vi "GetVibrationChannelProperties.vi"(10 "all channels":T2[](array[typedef]), 11 "channel":T2) -> (2 "TDMS properties":T1[](array[typedef]))   [LabVIEW 2017, in "Tdms.lvlib"]
doc: "Returns TDMS properties that define how a waveform channel works. Use the TDMS Set Properties function to write these properties to a TDMS file that contains data from the channel."
uses:
  <vilib>/addons/InsightCM/Utilities/Tdms/Tdms.lvlib
  <vilib>/addons/InsightCM/MessageBus/Base/controls/R2_Channel.ctl
  <vilib>/addons/InsightCM/MessageBus/Base/controls/KeyValuePair.ctl
  <vilib>/addons/InsightCM/MessageBus/Base/controls/Metric.ctl
  <vilib>/addons/InsightCM/Utilities/Tdms/controls/Property.ctl
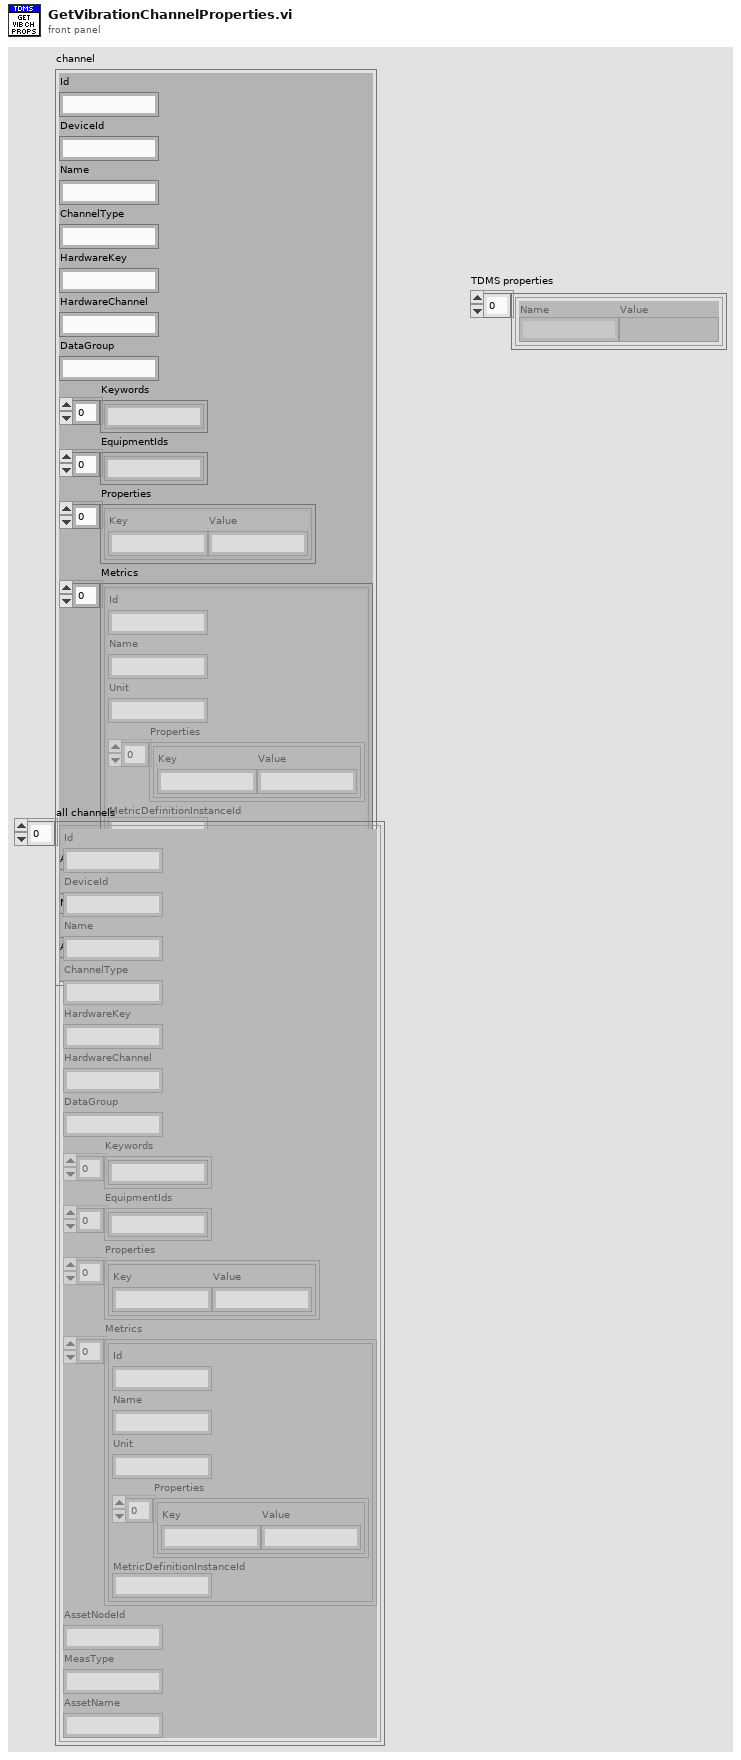
[diagram p1: front panel]
types:
  T1 = typedef "Tdms.lvlib/Property.ctl" = cluster{"Name":string, "Value":variant}
  T2 = typedef "R2_Channel.ctl" = cluster{"Id":string, "DeviceId":string, "Name":string, "ChannelType":string, "HardwareKey":string, "HardwareChannel":string, "DataGroup":string, "Keywords":string[], "EquipmentIds":string[], "Properties":T3[], "Metrics":T4[], "AssetNodeId":string, "MeasType":string, "AssetName":string}
  T3 = typedef "KeyValuePair.ctl" = cluster{"Key":string, "Value":string}
  T4 = typedef "Metric.ctl" = cluster{"Id":string, "Name":string, "Unit":string, "Properties":T3[], "MetricDefinitionInstanceId":string}
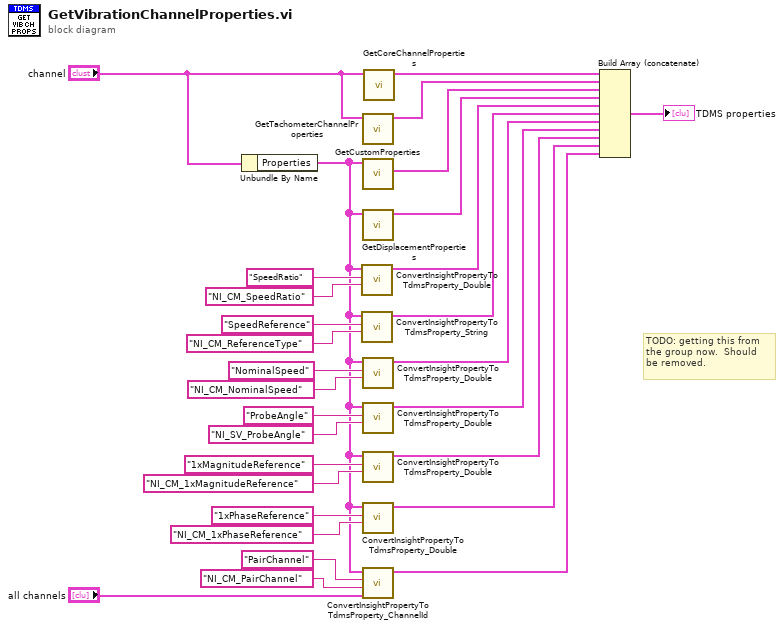
[diagram p0: block diagram]
diagram:
  # "TODO: getting this from\nthe group now.  Should\nbe removed."
  n1 = Unbundle By Name("channel") -> ("Properties"=w3:T3[])
  n2 = call <vilib>:"ConvertInsightPropertyToTdmsProperty_Double.vi"("Tdms Property Name"="NI_CM_SpeedRatio" ("Name"), "Insight Property Name"="SpeedRatio" ("Name"), "Insight Properties"=w3) -> ("Tdms Properties"=w2:T1[])  [unwired: 8 in]
  n3 = call <vilib>:"ConvertInsightPropertyToTdmsProperty_String.vi"("Tdms Property Name"="NI_CM_ReferenceType" ("Name"), "Insight Property Name"="SpeedReference" ("Name"), "Insight Properties"=w3) -> ("Tdms Properties"=w14:T1[])  [unwired: 8 in]
  n4 = call <vilib>:"GetTachometerChannelProperties.vi"("Channel"="channel") -> ("Tachometer Properties"=w7:T1[])  [unwired: 10 in]
  n5 = call <vilib>:"GetCustomProperties.vi"("Properties"=w3) -> ("Tdms Properties"=w6:T1[])  [unwired: 10 in]
  n6 = call <vilib>:"GetDisplacementProperties.vi"("channel properties"=w3) -> ("tdms properties"=w1:T1[])  [unwired: 10 in]
  n7 = call <vilib>:"ConvertInsightPropertyToTdmsProperty_Double.vi"("Tdms Property Name"="NI_CM_NominalSpeed" ("Name"), "Insight Property Name"="NominalSpeed" ("Name"), "Insight Properties"=w3) -> ("Tdms Properties"=w13:T1[])  [unwired: 8 in]
  n8 = call <vilib>:"ConvertInsightPropertyToTdmsProperty_Double.vi"("Tdms Property Name"="NI_SV_ProbeAngle" ("Name"), "Insight Property Name"="ProbeAngle" ("Name"), "Insight Properties"=w3) -> ("Tdms Properties"=w12:T1[])  [unwired: 8 in]
  n9 = call <vilib>:"ConvertInsightPropertyToTdmsProperty_Double.vi"("Tdms Property Name"="NI_CM_1xMagnitudeReference" ("Name"), "Insight Property Name"="1xMagnitudeReference" ("Name"), "Insight Properties"=w3) -> ("Tdms Properties"=w11:T1[])  [unwired: 8 in]
  n10 = call <vilib>:"ConvertInsightPropertyToTdmsProperty_Double.vi"("Tdms Property Name"="NI_CM_1xPhaseReference" ("Name"), "Insight Property Name"="1xPhaseReference" ("Name"), "Insight Properties"=w3) -> ("Tdms Properties"=w10:T1[])  [unwired: 8 in]
  n11 = call <vilib>:"ConvertInsightPropertyToTdmsProperty_ChannelId.vi"("Insight Channels"="all channels", "Tdms Property Name"="NI_CM_PairChannel" ("Name"), "Insight Property Name"="PairChannel" ("Name"), "Insight Properties"=w3) -> ("Tdms Properties"=w4:T1[])  [unwired: 7 in]
  n12 = call <vilib>:"GetCoreChannelProperties.vi"("Channel"="channel") -> ("Tdms Properties"=w8:T1[])  [unwired: 10 in]
  n13 = Build Array (concatenate)(w8, w7, w6, w1, w2, w14, w13, w12, w11, w10, w4) -> (→"TDMS properties":T1[])
